vi "TSM SSC Scope Pins to Sessions.vi"(0 "TSM context":T3, 5 "Pins":string[](array[string]), 7 "Site Numbers":i32[](array[numeric]), 11 "error in":errorcluster) -> (4 "TSM Scope Out":T1, 15 "error out":errorcluster)   [LabVIEW 2020]
doc: "Populates the TSM SSC Scope cluster for the specified pin(s) and pin group(s)."
uses:
  <vilib>/NI_TestStand_SemiconductorModule/NI_TestStand_Semiconductor_Module.lvlibp/PinMap/General/SemiconductorModuleContext.ctl
  TSM SSC Scope.ctl
  <vilib>/NI_TestStand_SemiconductorModule/NI_TestStand_Semiconductor_Module.lvlibp/PinMap/PinQueryContext/MultiplePinMultipleSessionQueryContext/MultiplePinMultipleSessionQueryContext.lvclass
  C:/Program Files/National Instruments/LabVIEW 2020/vi.lib/NI_TestStand_SemiconductorModule/NI_TestStand_Semiconductor_Module.lvlibp/PinMap/PinQueryContext/PinQueryContext.lvclass
  SSC Scope.ctl
  <vilib>/NI_TestStand_SemiconductorModule/NI_TestStand_Semiconductor_Module.lvlibp/PinMap/Scope/PinsToNISCOPESessions.vi
  <vilib>/NI_TestStand_SemiconductorModule/NI_TestStand_Semiconductor_Module.lvlibp
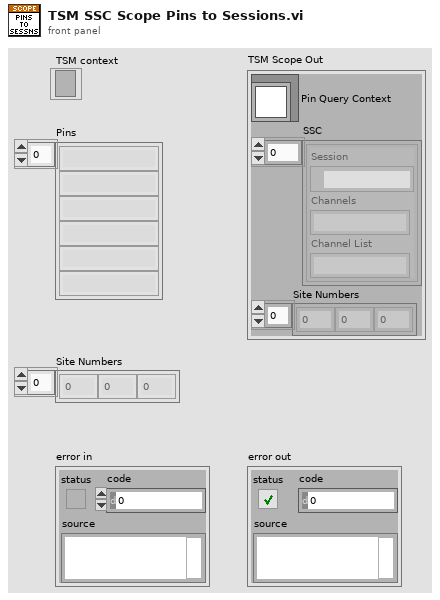
[diagram p1: front panel]
types:
  T1 = typedef "TSM SSC Scope.ctl" = cluster{"Pin Query Context":refnum<class "MultiplePinMultipleSessionQueryContext.lvclass">, "SSC":T2[], "Site Numbers":i32[]}
  T2 = typedef "SSC Scope.ctl" = cluster{"Session":refnum<k15>, "Channels":string, "Channel List":string}
  T3 = typedef "NI_TestStand_Semiconductor_Module.lvlibp/SemiconductorModuleContext.ctl" = refnum<k7>
  T4 = cluster{"Instrument Session":refnum<k15>, "Channel List":string, "spreadsheet string":string}[]
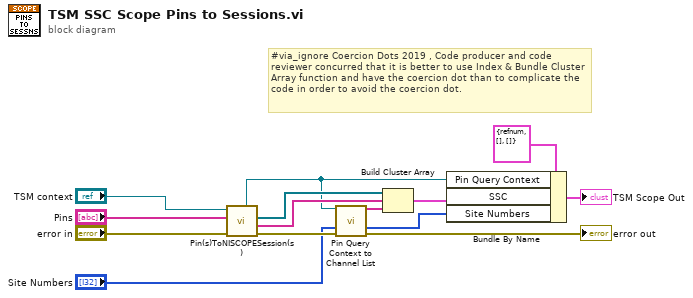
[diagram p0: block diagram]
diagram:
  # "#via_ignore Coercion Dots 2019 , Code producer and code reviewer concurred that it is better to use Index & Bundle Cluster Array function and have the coercion dot than to complicate the code in order to avoid the coercion dot."
  n1 = call-poly <vilib>:"Pin(s)ToNISCOPESession(s).vi"("error in (no error)"="error in", "Pins"="Pins", "Semiconductor Module Context"="TSM context") -> ("error out"=w11:errorcluster, "Channel Lists"=w9:string[], "Instrument Sessions"=w10:refnum<k15>[], "Pin Query Context"=w6:refnum<class "MultiplePinMultipleSessionQueryContext.lvclass">)  [unwired: 4 in, 1 out]
  n2 = call "Pin Query Context to Channel List.vi"("Pin Query Context"=w6, "Site Numbers In"="Site Numbers", "error in"=w11) -> ("Per-Session Channel List"=w5:string[], "Site Numbers Out"=w1:i32[], "error out"=→"error out":errorcluster)  [unwired: 9 in, 1 out]
  n3 = Build Cluster Array(w10, w9, w5) -> (w8:T4)
  n4 = Bundle By Name(cluster=T1 {"Pin Query Context"=refnum, "SSC"=[], "Site Numbers"=[]} ("Scope - Multiple Sessions Info"), "Pin Query Context"=w6, "SSC"=w8, "Site Numbers"=w1) -> (→"TSM Scope Out":T1)
